vi "PCIe_BandWidth(CuLab).vi"() -> ()   [LabVIEW 2020]
doc: "This benchmark is designed to demonstrate execution performance improvement when executing FFT and IFFT operations on a GPU."
uses:
  893085e6-138a-4d68-af2c-42f6574c691e.vi
  15a52568-f626-485c-809b-6783e4cb849b.vi
  <vilib>/Utility/High Resolution Relative Seconds.vi
  <vilib>/Ngene/CuLab - GPU Accelerated Toolkit/Toolkit/Low_Level/Tensor_Classes/T_Children/T1D/T1D_Children/T1D_U8/Create_Push.vi
  <vilib>/Ngene/CuLab - GPU Accelerated Toolkit/Toolkit/Low_Level/Tensor_Classes/T_Children/T1D/T1D_Children/T1D_U8/Push.vi
  <vilib>/Ngene/CuLab - GPU Accelerated Toolkit/Toolkit/Low_Level/Tensor_Classes/T_Children/T1D/T1D_Children/T1D_U8/Pull.vi
  <vilib>/Ngene/CuLab - GPU Accelerated Toolkit/Toolkit/CuLab.lvlib
  <vilib>/Ngene/CuLab - GPU Accelerated Toolkit/Toolkit/Low_Level/Tensor_Classes/T_Children/T1D/T1D_Children/T1D_U8/T1D_U8.lvclass
  <vilib>/Analysis/NI_AALBase.lvlib
panel:
  out "Max BW":dbl[](array[numeric])=[5320605525.457515, 4091935287.7213206, 2314591607.020676] format="%#_3pB/s"
  out "BW(BiDir)":dbl[](array[numeric])=[42935011.010134175, 83762779.00228798, 204800005.1736833, 387328520.7130382, 659315894.1713425, 1023999886.1700423, 1051942252.1052823, 1336106047.5285428, 1634823799.8346186, 1800439549.240135, 1874297971.7070773, 2060171916.8922012, 2094481534.331993, 2199165804.019033, 2145328022.971457, 2068241856.7917824, 2175155100.902325, 2167046005.8175178, 2314591607.020676] format="%_3p"
  out "BW(Push)":dbl[](array[numeric])=[111912561.56658754, 152267610.56309456, 447650246.26635015, 827475136.3086066, 502576730.09849614, 1527645455.4852219, 2861834092.513641, 3360820315.569827, 3813003657.0247936, 3939053387.9506445, 3890098302.3806424, 4983726246.169832, 5316648492.713752, 4600404731.13033, 5062680224.725092, 4954182741.205939, 4640326370.323135, 4733585075.86405, 5320605525.457515] format="%_3p"
  out "BW(Pull)":dbl[](array[numeric])=[93515984.25291894, 175042708.441015, 360881085.47123337, 682666435.5596689, 1149754143.496277, 1785722280.578998, 2047999772.3400846, 2422772605.076155, 2794712117.895021, 2978909067.6425905, 2810065656.589091, 3223164548.5609536, 3366485274.261984, 3481255781.236867, 3488458107.0141435, 3691580020.4726043, 3653843461.2527, 3849707093.7121186, 4091935287.7213206] format="%_3p"
  out "Iteration":i32=49
  out "Data Size (Bytes)":i32=268435456 format="%_3p"
  out "GPU Model":string="NVIDIA GeForce GTX 1650 Ti"
  out "CPU Model":string="Intel(R) Core(TM) i7-10750H CPU @ 2.60GHz  "
  in  "No. of Repetitions":i32=50
  in  "Data Size Stop (2^N)":i32=28
  in  "Data Size Start (2^N)":i32=10
  out "Data Sizes":i32[](array[numeric])=[1024, 2048, 4096, 8192, 16384, 32768, 65536, 131072, 262144, 524288, 1048576, 2097152, 4194304, 8388608, 16777216, 33554432, 67108864, 134217728, 268435456] format="%#_3pB"
  out "BW(Bytes/sec)":cluster{i32[], "FFT mean Exec Time":dbl[]}[](graph)=[{[1024, 2048, 4096, 8192, 16384, 32768, 65536, 131072, 262144, 524288, 1048576, 2097152, 4194304, 8388608, 16777216, 33554432, 67108864, 134217728, 268435456], "FFT mean Exec Time"=[111912561.56658754, 152267610.56309456, 447650246.26635015, 827475136.3086066, 502576730.09849614, 1527645455.4852219, 2861834092.513641, 3360820315.569827, 3813003657.0247936, 3939053387.9506445, 3890098302.3806424, 4983726246.169832, 5316648492.713752, 4600404731.13033, 5062680224.725092, 4954182741.205939, 4640326370.323135, 4733585075.86405, 5320605525.457515]}, {[1024, 2048, 4096, 8192, 16384, 32768, 65536, 131072, 262144, 524288, 1048576, 2097152, 4194304, 8388608, 16777216, 33554432, 67108864, 134217728, 268435456], "FFT mean Exec Time"=[93515984.25291894, 175042708.441015, 360881085.47123337, 682666435.5596689, 1149754143.496277, 1785722280.578998, 2047999772.3400846, 2422772605.076155, 2794712117.895021, 2978909067.6425905, 2810065656.589091, 3223164548.5609536, 3366485274.261984, 3481255781.236867, 3488458107.0141435, 3691580020.4726043, 3653843461.2527, 3849707093.7121186, 4091935287.7213206]}, {[1024, 2048, 4096, 8192, 16384, 32768, 65536, 131072, 262144, 524288, 1048576, 2097152, 4194304, 8388608, 16777216, 33554432, 67108864, 134217728, 268435456], "FFT mean Exec Time"=[42935011.010134175, 83762779.00228798, 204800005.1736833, 387328520.7130382, 659315894.1713425, 1023999886.1700423, 1051942252.1052823, 1336106047.5285428, 1634823799.8346186, 1800439549.240135, 1874297971.7070773, 2060171916.8922012, 2094481534.331993, 2199165804.019033, 2145328022.971457, 2068241856.7917824, 2175155100.902325, 2167046005.8175178, 2314591607.020676]}]
  # "Overview: CPU to GPU (PCIe) Bandwidth Test"
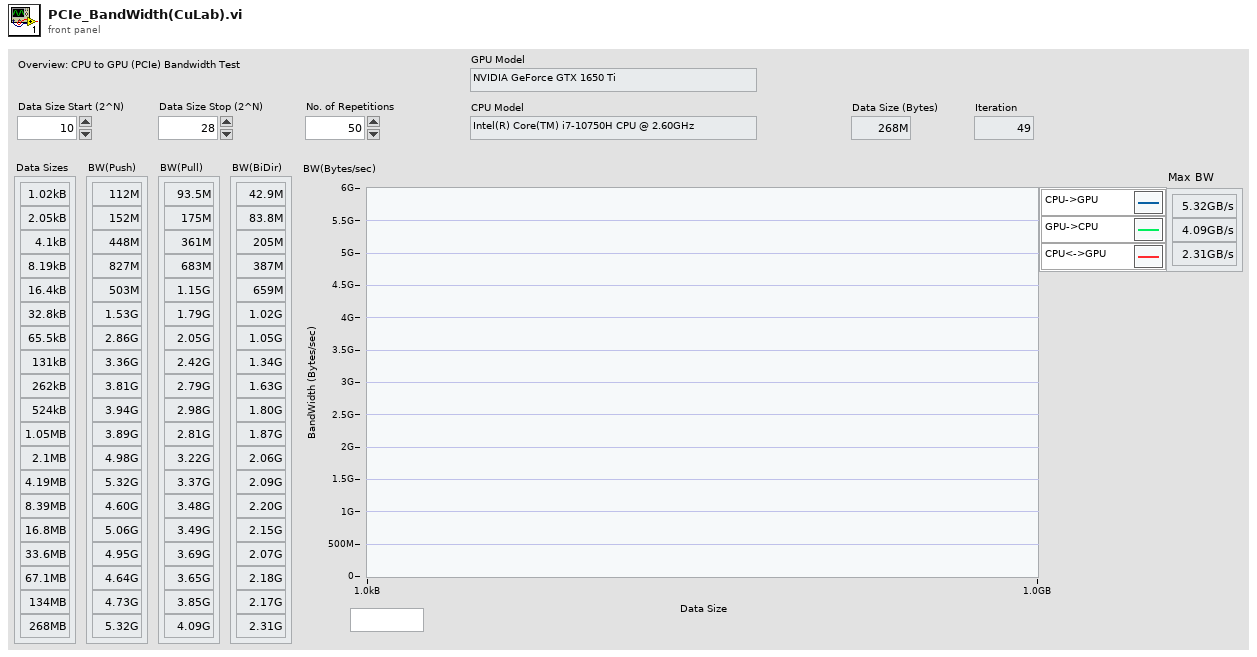
[diagram p1: front panel]
types:
  T1 = typedef "CuLab.lvlib/Properties.ctl" = cluster{"Index":i32, "Name":string}
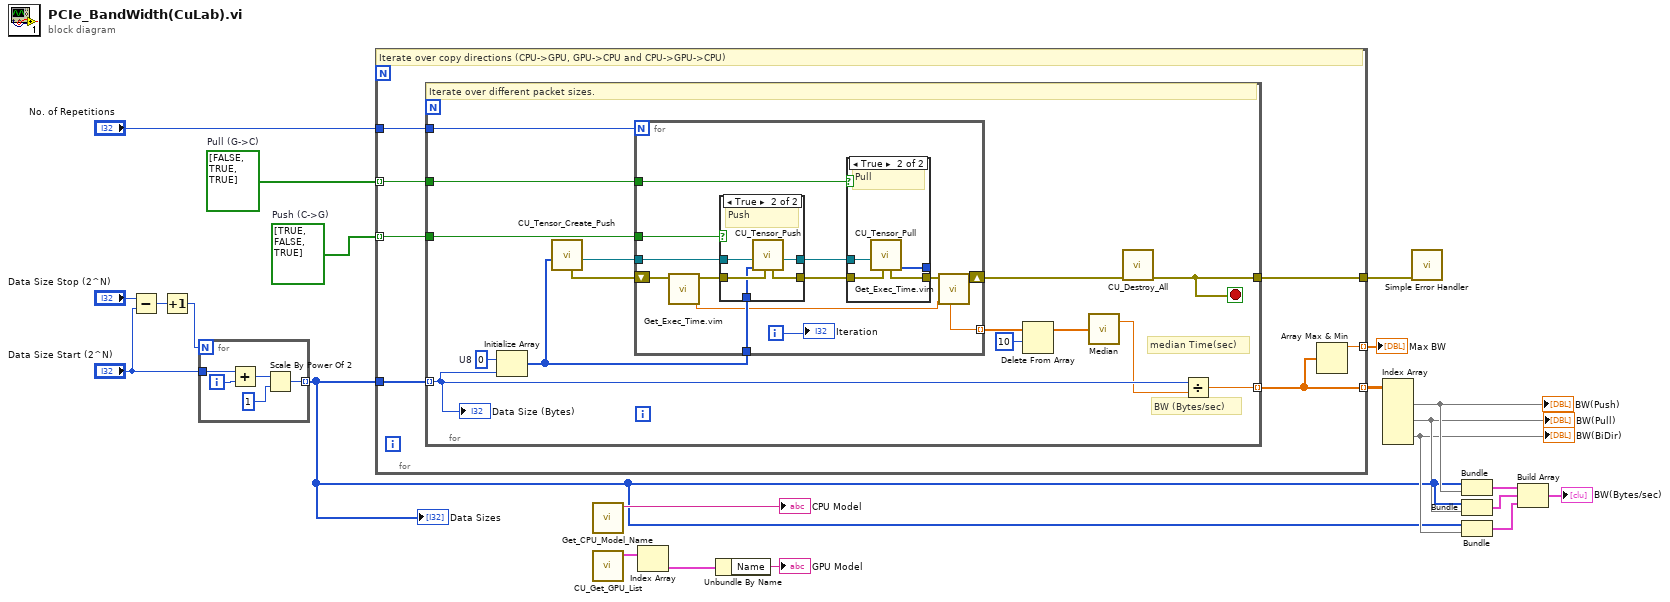
[diagram p0: block diagram]
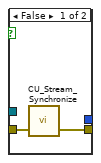
[diagram p2: hidden frame]
diagram:
  w8 = bool[] [FALSE, TRUE, TRUE]  # Pull (G->C)
  w9 = bool[] [TRUE, FALSE, TRUE]  # Push (C->G)
  n1 = Subtract(x="Data Size Stop (2^N)", y="Data Size Start (2^N)") -> (x-y=w19:i32)
  n2 = Increment(x=w19) -> (x+1=w18:i32)
  n3 = for {
    N: w18 -> [_]
    tunnel: "Data Size Start (2^N)" -> [w27]
    tunnel: [w23] -> w1 mode=indexing
    i -> [w26]
    n4 = Add(x=w27, y=w26) -> (x+y=w25:i32)
    n5 = Scale By Power Of 2(n=w25, x=1) -> (x*2^n=w23:i32)
  }
  "Data Sizes" <- w1
  n6 = for {
    tunnel: "No. of Repetitions" -> [w34]
    tunnel: [w33] -> w15
    tunnel: w1 -> [w32]
    tunnel: [w29] -> w10 mode=indexing
    tunnel: w9 -> [w31] mode=indexing
    tunnel: w8 -> [w30] mode=indexing
    tunnel: [w28] -> w2 mode=indexing
    # "Iterate over copy directions (CPU->GPU, GPU->CPU and CPU->GPU->CPU)"
    n7 = for {
      tunnel: [w46] -> w33
      tunnel: [w40] -> w29 mode=indexing
      tunnel: w32 -> [w39] mode=indexing
      tunnel: w34 -> [w41]
      tunnel: w31 -> [w43]
      tunnel: w30 -> [w42]
      stop <- w46 stop-if-true
      w45 = u8 0  # U8
      # "median Time(sec)"
      # "BW (Bytes/sec)"
      # "Iterate over different packet sizes."
      n8 = Initialize Array(w45, w39) -> (w47:u8[])
      n9 = call-poly <vilib>:"CU_Tensor_Create_Push.vi"("T1D_U8_Data"=w47) -> ("T1D_U8 out"=w49:refnum<class "T1D_U8.lvclass">, "error out"=w44:errorcluster)  [unwired: 9 in]
      n10 = for {
        N: w41 -> [_]
        tunnel: w49 -> [w62]
        tunnel: w47 -> [w59]
        shift-right: [w53] -> w48
        shift-left: w44 -> [w61]
        tunnel: w43 -> [w56]
        tunnel: w42 -> [w55]
        tunnel: [w51] -> w37 mode=indexing
        i -> [w50]
        n11 = call "Get_Exec_Time.vim"("error in (no error)"=w61) -> ("T(n)"=w52:dbl, "error out"=w54:errorcluster)  [unwired: 6 in, 1 out]
        n12 = case shown="True" w56 {
          tunnel: w62 -> [w69 w75]
          tunnel: w54 -> [w70 w74]
          tunnel: w59 -> [_ w73]
          tunnel: [w70 w72] -> w58
          tunnel: [w69 w71] -> w57
          frame False {
          }
          frame True {
            # "Push"
            n13 = call-poly <vilib>:"CU_Tensor_Push.vi"("error in (no error)"=w74, "T1D_U8_Data"=w73, "T1D_U8 in"=w75) -> ("T1D_U8 out"=w71:refnum<class "T1D_U8.lvclass">, "error out"=w72:errorcluster)  [unwired: 7 in]
          }
        }
        n14 = case shown="True" w55 {
          tunnel: [w63 w68] -> w60
          tunnel: w58 -> [w64 w67]
          tunnel: w57 -> [_ w66]
          tunnel: [_ w65] -> _
          frame False {
            n15 = call <vilib>:"CU_Stream_Synchronize.vi"("error in (no error)"=w64) -> ("error out"=w63:errorcluster)  [unwired: 10 in]
          }
          frame True {
            # "Pull"
            n16 = call-poly <vilib>:"CU_Tensor_Pull.vi"("error in (no error)"=w67, "T1D_U8 in"=w66) -> ("Dest out"=w65:u8[], "error out"=w68:errorcluster)  [unwired: 7 in, 1 out]
          }
        }
        n17 = call "Get_Exec_Time.vim"("T(n-1)"=w52, "error in (no error)"=w60) -> ("error out"=w53:errorcluster, "dT"=w51:dbl)  [unwired: 5 in, 1 out]
        "Iteration" <- w50
      }
      n18 = Delete From Array(array=w37, length=10) -> (array with subset deleted=w36:dbl[])  [unwired: 1 in, 1 out]
      n19 = call <vilib>:"Median.vi"("X"=w36) -> ("median"=w38:dbl)  [unwired: 1 out]
      n20 = call <vilib>:"CU_Destroy_All.vi"("error in"=w48) -> ("error out"=w46:errorcluster)  [unwired: 10 in]
      n21 = Divide(x=w39, y=w38) -> (x/y=w40:dbl)
      "Data Size (Bytes)" <- w39
    }
    n22 = Array Max & Min(array=w29) -> (max value=w28:dbl)  [unwired: 3 out]
  }
  "Max BW" <- w2
  n23 = call "Get_CPU_Model_Name.vi"() -> ("CPU Model"=→"CPU Model":string)  [unwired: 11 in]
  n24 = call <vilib>:"CU_Get_GPU_List.vi"() -> ("Devices"=w13:T1[])  [unwired: 10 in, 1 out]
  n25 = Index Array(array=w13) -> (element=w12:T1)  [unwired: 1 in]
  n26 = Unbundle By Name(w12) -> ("Name"=→"GPU Model":string)
  n27 = Index Array(array=w10) -> (element #1=w5:dbl[], element #2=w4:dbl[], element #3=w3:dbl[])  [unwired: 6 in]
  "BW(Pull)" <- w4
  "BW(Push)" <- w5
  "BW(BiDir)" <- w3
  n28 = call <vilib>:"Simple Error Handler.vi"("error in (no error)"=w15) -> ()  [unwired: 4 in, 5 out]
  n29 = Bundle(w1, w5) -> (w7:cluster{i32[], dbl[]})  [unwired: 1 in]
  n30 = Bundle(w1, w4) -> (w22:cluster{i32[], dbl[]})  [unwired: 1 in]
  n31 = Bundle(w1, w3) -> (w6:cluster{i32[], dbl[]})  [unwired: 1 in]
  n32 = Build Array(w7, w22, w6) -> (→"BW(Bytes/sec)":cluster{i32[], dbl[]}[])
